vi "Save Collimation Data in EQdb.vi"(0 "Records":T1, 1 "Server (API default)":string, 2 "Write direct to nEQdb (F)":bool, 3 "Process Sub Step":string(combo), 5 "Process to LEQdb":bool, 7 "ITAR":bool, 9 "TestNumber":i32, 11 "error in (no error)":errorcluster, 12 "Database (API default)":string, 13 "XML save directory (API default)":string) -> (4 "XML path":string, 6 "Database primary key":i32, 15 "error out":errorcluster)   [LabVIEW 2018]
doc: "This VI uses the nEQdbAPI DLL to convert the Device Data cluster into an XML file to be imported into the LQEdb.\n\nFor the \"Process to LEQdb\" boolean, TRUE means to process the XML file inside the LEQdb, instead of just storing the contents.\n\nThe \"Calculations to do when saving\" input enables the selected standard calculations in the nEQdb API. These calculations use data points in the various data structures that may have been written to previously, and enabling these calculations will overwrite those data points. If any specific calculation is enabled but does not have data to exectute, nothing will happen; consult external documentation if a calculation is enabled here but doesn't appear to be doing anything."
uses:
  State data/Records.ctl
  C:/Program Files (x86)/National Instruments/LabVIEW 2018/user.lib/nEQdb_DLL/NEQdbAPI.dll
  Program Files (x86)/National Instruments/LabVIEW 2018/user.lib/nEQdb_DLL/NEQdbAPI.dll
  <vilib>/Utility/error.llb/Clear Errors.vi
  <userlib>/nLight Error Handling/Log any errors.vi
panel:
  out "xmlId":i64
  # "TRUE means to process the XML file inside the LEQdb, instead of just storing the contents"
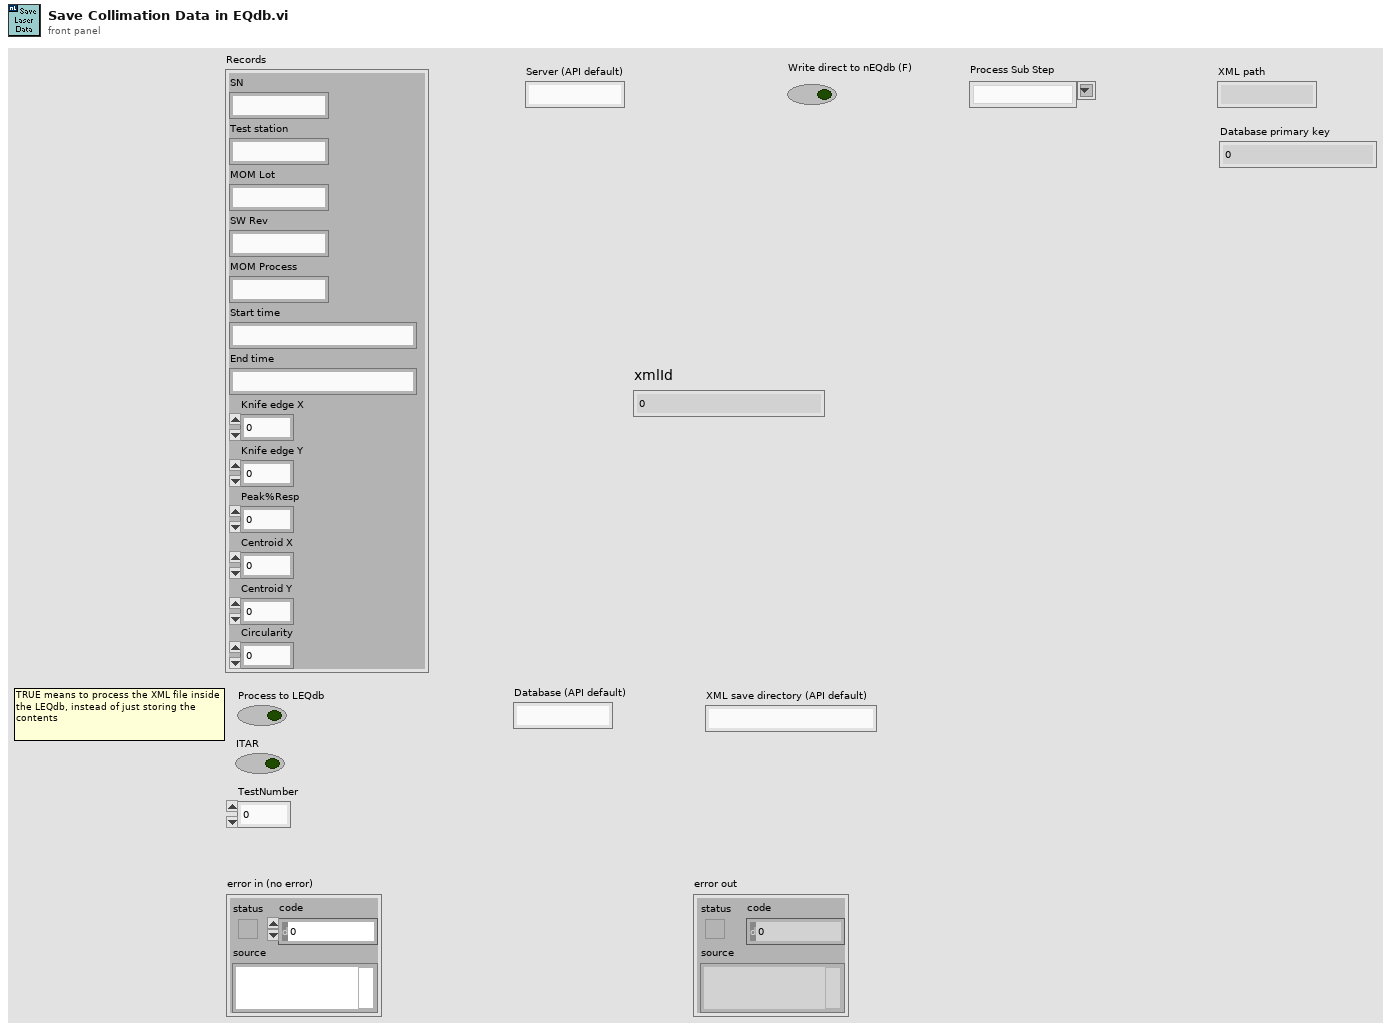
[diagram p1: front panel]
types:
  T1 = typedef "Records.ctl" = cluster{"SN":string, "Test station":string, "MOM Lot":string, "SW Rev":string, "MOM Process":string, "Start time":string, "End time":string, "Knife edge X":dbl, "Peak%Resp":dbl, "Centroid X":dbl, "Knife edge Y":dbl, "Centroid Y":dbl, "Circularity":dbl}
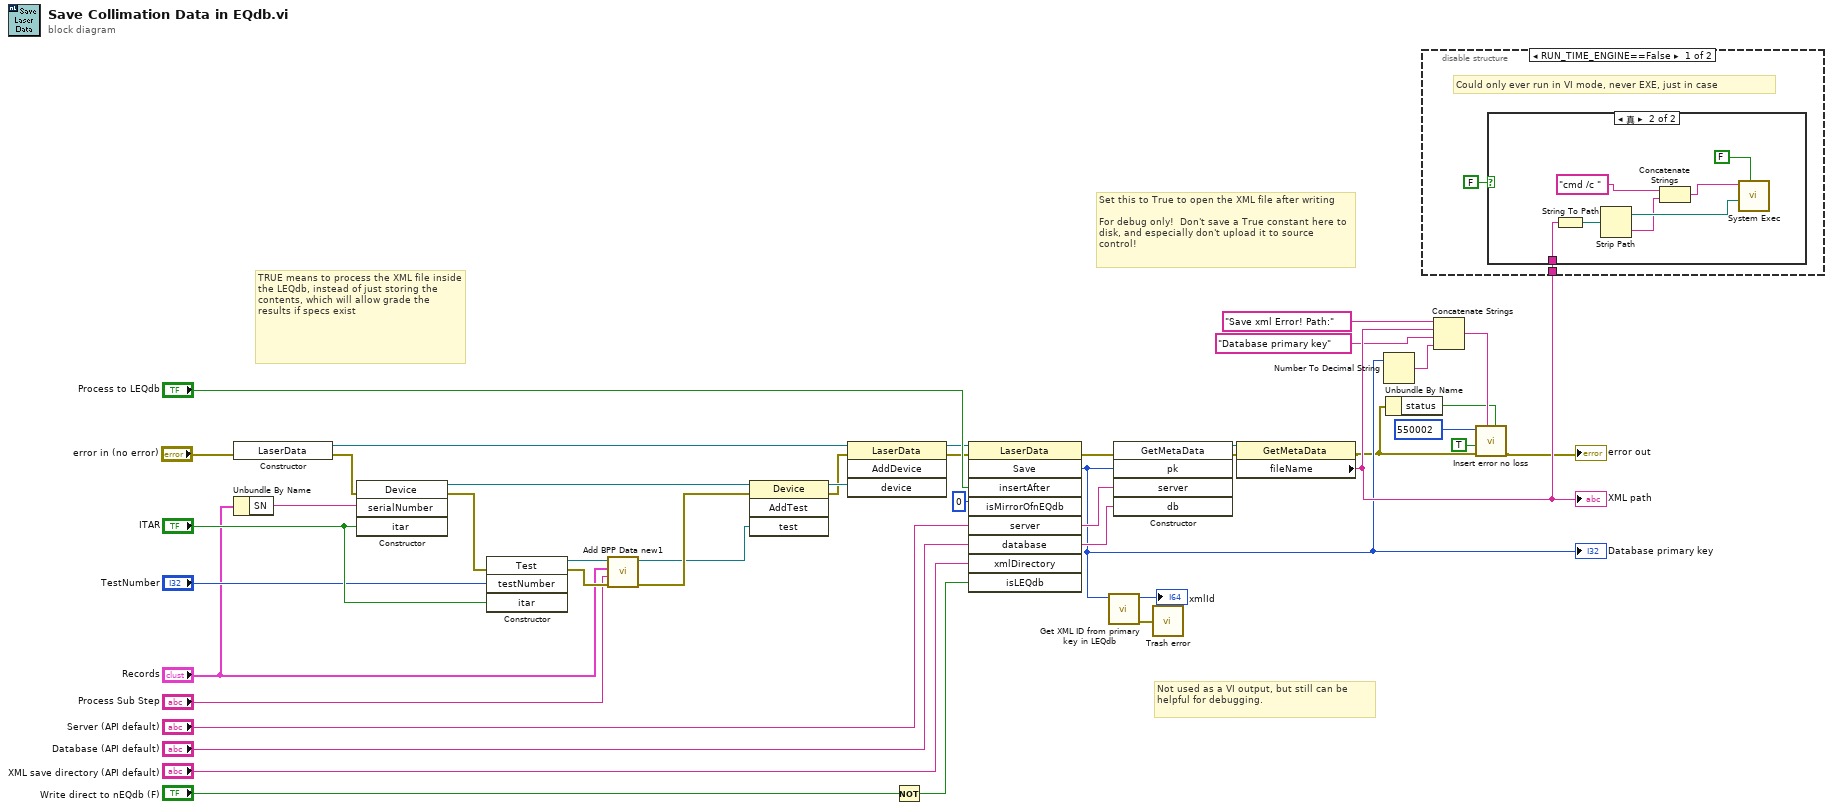
[diagram p0: block diagram]
diagram:
  # "Not used as a VI output, but still can be helpful for debugging."
  # "Set this to True to open the XML file after writing\n\nFor debug only!  Don't save a True constant here to disk, and especially don't upload it to source control!"
  # "TRUE means to process the XML file inside the LEQdb, instead of just storing the contents, which will allow grade the results if specs exist"
  n1 = constructor class="LaserData"(error in="error in (no error)") -> (reference out=w36:refnum<k24>, error out=w41:errorcluster)  [unwired: 2 in, 1 out]
  n2 = Unbundle By Name("Records") -> ("SN"=w14:string)
  n3 = constructor class="Device"(error in=w41, "serialNumber"=w14, "itar"="ITAR") -> (reference out=w40:refnum<k24>, error out=w39:errorcluster)  [unwired: 2 in, 3 out]
  n4 = constructor class="Test"(error in=w39, "testNumber"="TestNumber", "itar"="ITAR") -> (reference out=w18:refnum<k24>, error out=w19:errorcluster)  [unwired: 2 in, 3 out]
  n5 = call "Add BPP Data new1.vi"("error in (no error)"=w19, "Process Sub Step"="Process Sub Step", "Records"="Records", "Test in"=w18) -> ("error out"=w21:errorcluster, "Test out"=w20:refnum<k24>)  [unwired: 6 in]
  n6 = invoke class="Device" method="AddTest"(reference=w40, error in=w21, "test"=w20) -> (reference out=w38:refnum<k24>, error out=w37:errorcluster)  [unwired: 1 in, 2 out]
  n7 = invoke class="LaserData" method="AddDevice"(reference=w36, error in=w37, "device"=w38) -> (reference out=w25:refnum<k24>, error out=w24:errorcluster)  [unwired: 1 in, 2 out]
  n8 = Not(x="Write direct to nEQdb (F)") -> (.not. x?=w27:bool)
  n9 = invoke class="LaserData" method="Save"(reference=w25, error in=w24, "insertAfter"="Process to LEQdb", "isMirrorOfnEQdb"=0, "server"="Server (API default)", "database"="Database (API default)", "xmlDirectory"="XML save directory (API default)", "isLEQdb"=w27) -> (error out=w31:errorcluster, "Save"=w5:i32)  [unwired: 1 in, 7 out]
  "Database primary key" <- w5
  n10 = call <userlib>:"Get XML ID from primary key in LEQdb.vi"("Database primary key"=w5) -> ("error out"=w22:errorcluster, "xmlId"=→"xmlId":i64)  [unwired: 9 in]
  n11 = constructor class="GetMetaData"(error in=w31, "pk"=w5, "server"="Server (API default)", "db"="Database (API default)") -> (reference out=w32:refnum<k24>, error out=w33:errorcluster)  [unwired: 2 in, 4 out]
  n12 = call <userlib>:"Trash error.vi"("error in"=w22) -> ()  [unwired: 15 in]
  n13 = property class="GetMetaData"(reference=w32, error in=w33) -> (error out=w2:errorcluster, "fileName"=w8:string)  [unwired: 1 out]
  "XML path" <- w8
  n14 = Number To Decimal String(number=w5) -> (decimal integer string=w6:string)  [unwired: 1 in]
  n15 = Unbundle By Name(w2) -> ("status"=w1:bool)
  n16 = disable-structure shown="RUN_TIME_ENGINE==False" {
    disable-tunnel: w8 -> [w43 _]
    frame condition #0 (active) {
      # "Could only ever run in VI mode, never EXE, just in case"
      n17 = case shown="真" FALSE {
        tunnel: w43 -> [_ w50]
        frame False {
        }
        frame True {
          n18 = String To Path(string=w50) -> (path=w44:path)
          n19 = Strip Path(path=w44) -> (stripped path=w49:path, name=w46:string)
          n20 = Concatenate Strings("cmd /c " ("command line"), w46) -> (w45:string)
          n21 = call <vilib>:"System Exec.vi"("wait until completion? (T)"=FALSE, "working directory"=w49, "command line"=w45) -> ()  [unwired: 5 in, 4 out]
        }
      }
    }
    frame condition #1 {
    }
  }
  n22 = Concatenate Strings("Save xml Error! Path:" ("format string"), w8, "Database primary key" ("字符串"), w6) -> (w9:string)
  n23 = call <userlib>:"Insert error no loss.vi"("Add error? (T)"=w1, "error message"=w9, "error in (no error)"=w2, "Error = T, Warning = F (T)"=TRUE, "error code"=550002) -> ("error out"=→"error out":errorcluster)  [unwired: 4 in]
